vi "Close.vi"(8 "error in (no error)":errorcluster, 11 "Bus in":refnum<class "Bus.lvclass">) -> (0 "error out":errorcluster, 3 "Bus out":refnum<class "Bus.lvclass">)   [LabVIEW 2015, in "Bus.lvclass"]
doc: "Bus.lvclass:Close.vi\n\nThis is the template for the Close VI for the bus class.\n\nInstrument Communication Module Version 1.0\nJuly, 2017 Original Code Consulting David Thomson\n www.originalcode.com"
uses:
  Bus.lvclass
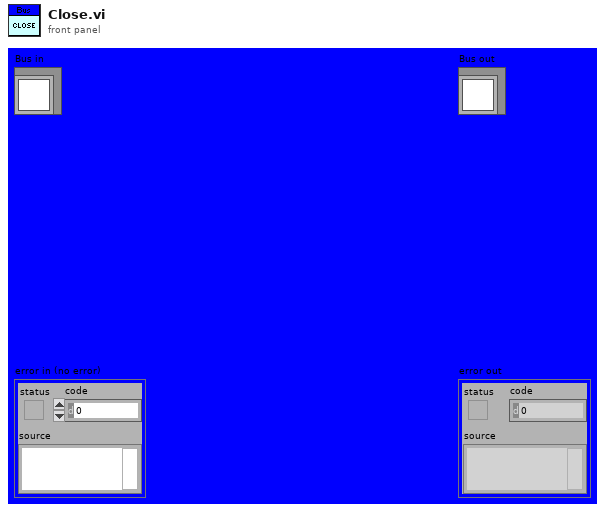
[diagram p1: front panel]
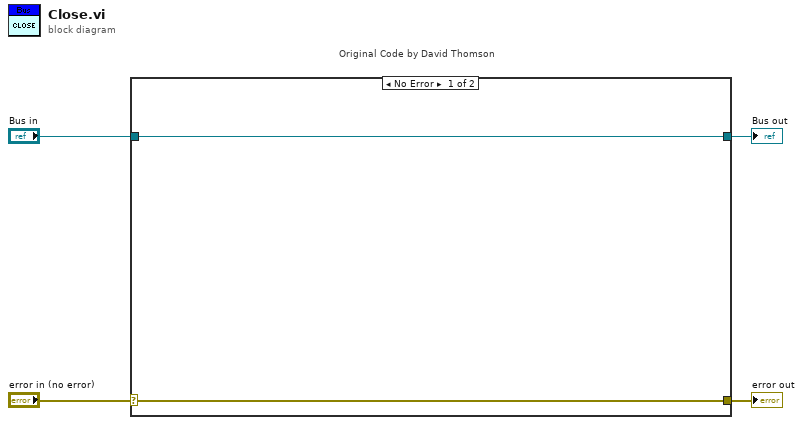
[diagram p0: block diagram]
diagram:
  n1 = case "Original Code by David Thomson" shown="No Error" "error in (no error)" {
    selector: "error in (no error)" -> [w5 w8]
    tunnel: [w5 w8] -> w3
    tunnel: [w6 w7] -> w1
    tunnel: "Bus in" -> [w6 w7]
    frame No Error {
    }
    frame Error {
    }
  }
  "error out" <- w3
  "Bus out" <- w1
